vi "CHD_SIM_SIM_Execute.vi"(6 "FPGA_Time_Seconds":dbl, 8 "error in (no error)":errorcluster) -> (0 "error out":errorcluster)   [LabVIEW 2019]
uses:
  <vilib>/Rock Robotics/WPI/ThirdParty/JAS_Junk/TrajLib/VI/Util_GetTime_U32.vi
  <vilib>/Rock Robotics/WPI/ThirdParty/JAS_Junk/TrajLib/Conv_Radians_Deg.vi
  <vilib>/Rock Robotics/WPI/ThirdParty/JAS_Junk/TrajLib/BatterySim_CalculateLoadedBatteryVoltage.vi
  <vilib>/Rock Robotics/WPI/ThirdParty/JAS_Junk/TrajLib/VI/Util_GetTime_U64.vi
  Differential_Drive_System/CHD_DRIVE_GLOBALS.vi
  CHD_SIM_SIM_Globals.vi
  <vilib>/Rock Robotics/WPI/ThirdParty/JAS_Junk/TrajLib/Trajectory_Library.lvlib
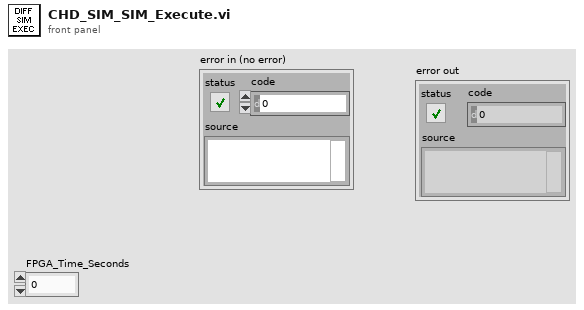
[diagram p1: front panel]
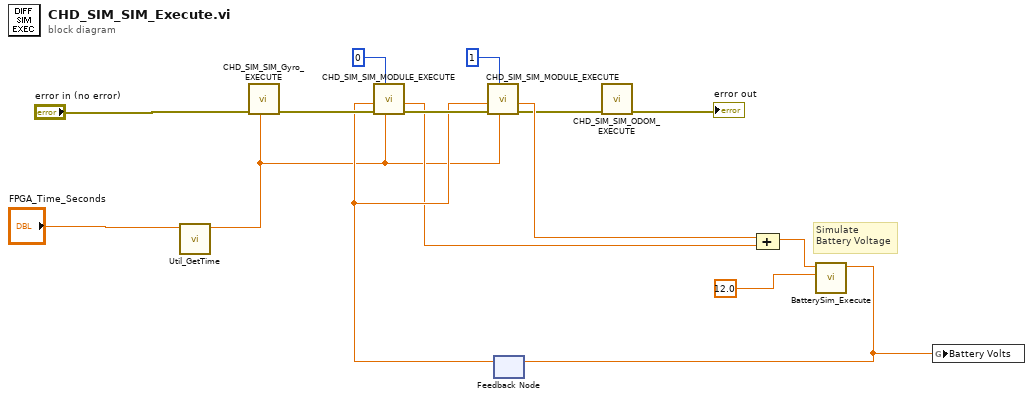
[diagram p0: block diagram]
diagram:
  # "Simulate\nBattery Voltage"
  n1 = call <vilib>:"Util_GetTime.vi"("Pass_Through_Time"="FPGA_Time_Seconds") -> ("FPGA_Time_Seconds"=w4:dbl)  [unwired: 8 in, 2 out]
  n2 = call "CHD_SIM_SIM_Gyro_EXECUTE.vi"("FPGA_Time_Seconds"=w4, "error in (no error)"="error in (no error)") -> ("error out"=w13:errorcluster)  [unwired: 9 in]
  n3 = feedback #1() -> (w7:dbl)  [unwired: 1 in]
  n4 = call "CHD_SIM_SIM_MODULE_EXECUTE.vi"("FPGA_Time_Seconds"=w4, "Module Index"=0, "error in (no error)"=w13, "Battery Voltage"=w7) -> ("error out"=w12:errorcluster, "Abs Current"=w5:dbl)  [unwired: 6 in]
  n5 = call "CHD_SIM_SIM_MODULE_EXECUTE.vi"("FPGA_Time_Seconds"=w4, "Module Index"=1, "error in (no error)"=w12, "Battery Voltage"=w7) -> ("error out"=w1:errorcluster, "Abs Current"=w6:dbl)  [unwired: 6 in]
  n6 = call "CHD_SIM_SIM_ODOM_EXECUTE.vi"("error in (no error)"=w1) -> ("error out"=→"error out":errorcluster)  [unwired: 10 in]
  n7 = Compound Arithmetic op=ADD(w6, w5) -> (w9:dbl)
  n8 = call <vilib>:"BatterySim_Execute.vi"("Nominal Battery Voltage"=12.0, "Current"=w9) -> ("Voltage"=w3:dbl)  [unwired: 9 in]
  n9 = feedback-in #1(w3) -> ()
  n10 = global write "CHD_SIM_SIM_Globals.vi" "Battery Volts"(w3) -> ()
